vi "FPGA - Download (ECAT).vi"(8 "error in (no error)":errorcluster, 11 "Node Ptr":u64 format="%.0x") -> (0 "error out":errorcluster)   [LabVIEW 2019, in "SEECD System Explorer.lvlib"]
uses:
  Type Defs/FPGA Target.ctl
  SEECD System Explorer.lvlib
panel:
  in  "Tag":string
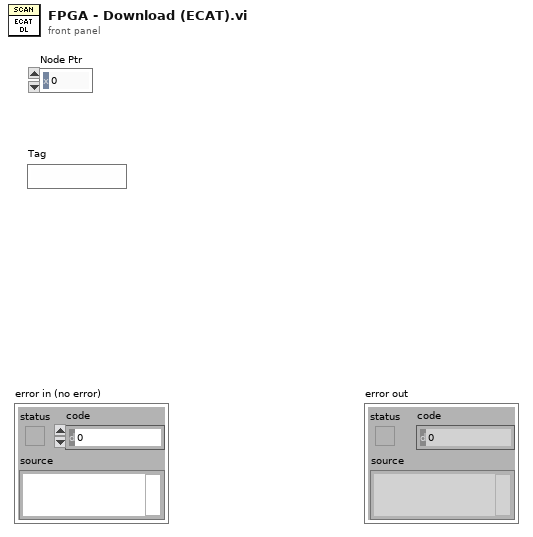
[diagram p1: front panel]
types:
  T1 = typedef "SEECD System Explorer.lvlib/FPGA Target.ctl" = enum16{"Local", "EtherCAT"}
  T2 = typedef "Custom Device API.lvlib/Custom Device Item Ref.ctl" = u64
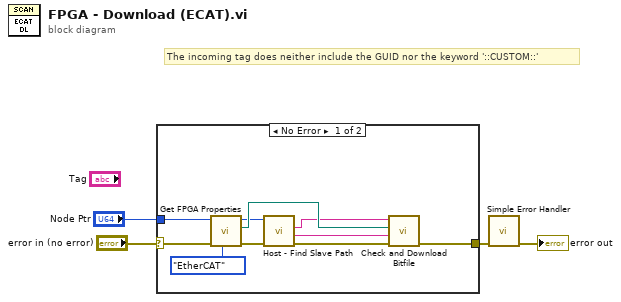
[diagram p0: block diagram]
diagram:
  # "The incoming tag does neither include the GUID nor the keyword '::CUSTOM::'"
  n1 = case shown="No Error" "error in (no error)" {
    selector: "error in (no error)" -> [w8 w15]
    tunnel: "Node Ptr" -> [w6 _]
    tunnel: [w7 w15] -> w2
    frame No Error {
      n2 = call "Get FPGA Properties.vi"("FPGA Target"=FPGA_Target."EtherCAT", "error in (no error)"=w8, "Item Ref in"=w6) -> ("error out"=w11:errorcluster, "Bitfile Path"=w13:path, "Item Ref out"=w12:T2)  [unwired: 5 in, 1 out]
      n3 = call "Host - Find Slave Path.vi"("error in (no error)"=w11, "Item Ref in"=w12) -> ("error out"=w10:errorcluster, "Target IP Address"=w5:string, "Slave Ref"=w9:string)  [unwired: 6 in, 1 out]
      n4 = call "Check and Download Bitfile.vi"("error in"=w10, "Target IP Address"=w5, "Bitfile Path"=w13, "Slave Ref"=w9) -> ("error out"=w7:errorcluster)  [unwired: 7 in]
    }
    frame Error {
    }
  }
  n5 = call <vilib>:"Simple Error Handler.vi"("error in (no error)"=w2) -> ("error out"=→"error out":errorcluster)  [unwired: 4 in, 4 out]
